vi "Drive Global.vi"() -> ()   [LabVIEW 2019]
panel:
  out "Pot values":T1={"Front Left Pot"=14.044803777629909, "Front Right Pot"=196.38893373729968, "Back Left Pot"=15.551006439084759, "Back Right Pot"=183.04899613827664}
  in  "Robot Width":dbl=23.0
  in  "Robot Length":dbl=23.0
  in  "Wheel Angle Offset":T2={"Front Left Offset"=132.6, "Front Right Offset"=117.3, "Back Left Offset"=123.8, "Back Right Offset"=151.7}
  in  "Rot point Y":dbl
  in  "Rot point X":dbl
  out "Yaw Pitch Roll":cluster{"Yaw":dbl, "Pitch":dbl, "Roll":dbl}={"Yaw"=-2707.91015625, "Pitch"=-0.087890625, "Roll"=5.0537109375}
  in  "Set Yaw Value":dbl
  in  "Set Yaw":bool
  in  "Drive Command":T3={"Y Command"=0.08661417322834646, "X Command"=0.031496062992125984, "Z Command"=-0.07874015748031496}
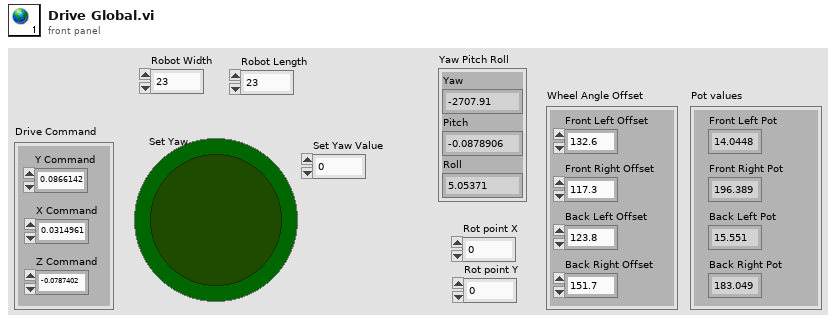
[diagram p1: front panel]
types:
  T1 = cluster{"Front Left Pot":dbl, "Front Right Pot":dbl, "Back Left Pot":dbl, "Back Right Pot":dbl}
  T2 = cluster{"Front Left Offset":dbl, "Front Right Offset":dbl, "Back Left Offset":dbl, "Back Right Offset":dbl}
  T3 = cluster{"Y Command":dbl, "X Command":dbl, "Z Command":dbl}
diagram:
